vi "Scatter.vi"() -> ()   [LabVIEW 2011]
uses:
  <vilib>/Heliosphere Research LLC/Advanced Plotting Toolkit/Advanced Plotting Toolkit.lvlib
  <vilib>/Heliosphere Research LLC/Advanced Plotting Toolkit/properties/Marker_Style.ctl
  <vilib>/Heliosphere Research LLC/Advanced Plotting Toolkit/typedefs/PlotColor.ctl
  <vilib>/Heliosphere Research LLC/Advanced Plotting Toolkit/properties/Marker.ctl
  <vilib>/Heliosphere Research LLC/Advanced Plotting Toolkit/properties/Line_Style.ctl
  <vilib>/Heliosphere Research LLC/Advanced Plotting Toolkit/properties/Line.ctl
  <vilib>/Heliosphere Research LLC/Advanced Plotting Toolkit/properties/Colormap_Map.ctl
  <vilib>/Heliosphere Research LLC/Advanced Plotting Toolkit/properties/Colormap_Scaling.ctl
  <vilib>/Heliosphere Research LLC/Advanced Plotting Toolkit/properties/Colormap.ctl
  <vilib>/Heliosphere Research LLC/Advanced Plotting Toolkit/properties/Display.ctl
  <vilib>/Heliosphere Research LLC/Advanced Plotting Toolkit/api_plotting/ScatterProperties.ctl
panel:
  in  "Line Appearance":T1={"Style"=enum."Automatic", "Color"=2147483647, "Width"=nan} {"Color" items=["Automatic"=2147483647, "Black"=0, "White"=16777215, "Red"=16711680, "Green"=2263842, "Blue"=255, "Cyan"=65535, "Magenta"=16711935, "Yellow"=16776960]}
  in  "Marker Appearance":T4={"Style"=enum."Automatic", "Color"=2147483647, "Size"=nan} {"Color" items=["Automatic"=2147483647, "Black"=0, "White"=16777215, "Red"=16711680, "Green"=2263842, "Blue"=255, "Cyan"=65535, "Magenta"=16711935, "Yellow"=16776960]}
  in  "Use Colormap Values":bool=TRUE
  in  "Use Areas":bool=TRUE
  out "Log Plot":picture
  # "Scatter Plots"
  # "A scatter plot displays any data available as X/Y pairs.\n\nIn addition to simply displaying markers, Scatter.vi allows you\nto convey information using the size and color of the markers.\nThe \"Areas\" and \"Colormap Values\" inputs allow you to\ncontrol these properties on a point-by-point basis.\n\nIn this example, the areas and colors are set according to the\npoints' distance from the origin, but any 1D data may be used\ninstead.  Use the boolean controls below to turn the areas\nand colors on and off.  You can also set basic properties like the\nmarker shape and outline using the property cluster."
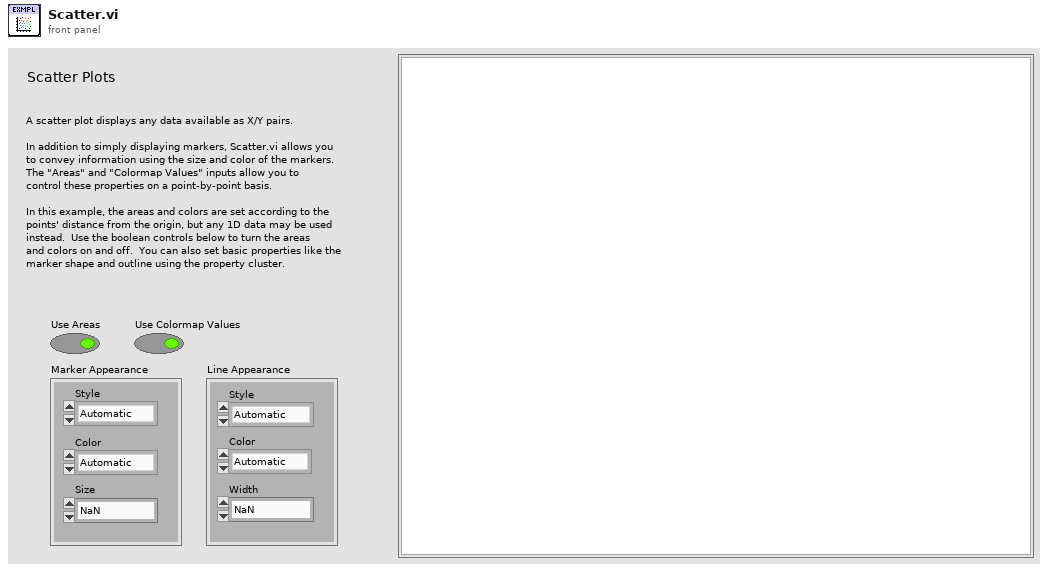
[diagram p1: front panel]
types:
  T1 = typedef "Advanced Plotting Toolkit.lvlib/Line.ctl" = cluster{"Style":T2, "Color":T3, "Width":sgl}
  T2 = typedef "Advanced Plotting Toolkit.lvlib/Line_Style.ctl" = enum16{"Automatic", "Solid", "Dashed", "Dotted", "Dash-dot", "Invisible"}
  T3 = typedef "Advanced Plotting Toolkit.lvlib/PlotColor.ctl" = u32
  T4 = typedef "Advanced Plotting Toolkit.lvlib/Marker.ctl" = cluster{"Style":T5, "Color":T3, "Size":dbl}
  T5 = typedef "Advanced Plotting Toolkit.lvlib/Marker_Style.ctl" = enum16{"Automatic", "Circle", "Square", "Triangle", "Diamond", "Star", "Invisible"}
  T6 = typedef "Advanced Plotting Toolkit.lvlib/ScatterProperties.ctl" = cluster{"Marker":T4, "Line":T1, "Colormap":T7, "Display":T10}
  T7 = typedef "Advanced Plotting Toolkit.lvlib/Colormap.ctl" = cluster{"Map":T8, "Value Min":dbl, "Value Max":dbl, "Scaling":T9, "Reverse":bool}
  T8 = typedef "Advanced Plotting Toolkit.lvlib/Colormap_Map.ctl" = enum16{"Automatic", "Rainbow", "Hot and Cold", "White-Black", "White-Blue", "White-Green", "White-Red", "Fire", "Water", "Earth", "Air", "Pastel", "Banded", "Stepped"}
  T9 = typedef "Advanced Plotting Toolkit.lvlib/Colormap_Scaling.ctl" = enum16{"Default"}
  T10 = typedef "Advanced Plotting Toolkit.lvlib/Display.ctl" = cluster{"Alpha":dbl, "Z Order":dbl}
  T11 = typedef "Advanced Plotting Toolkit.lvlib/PlotID.ctl" = i32
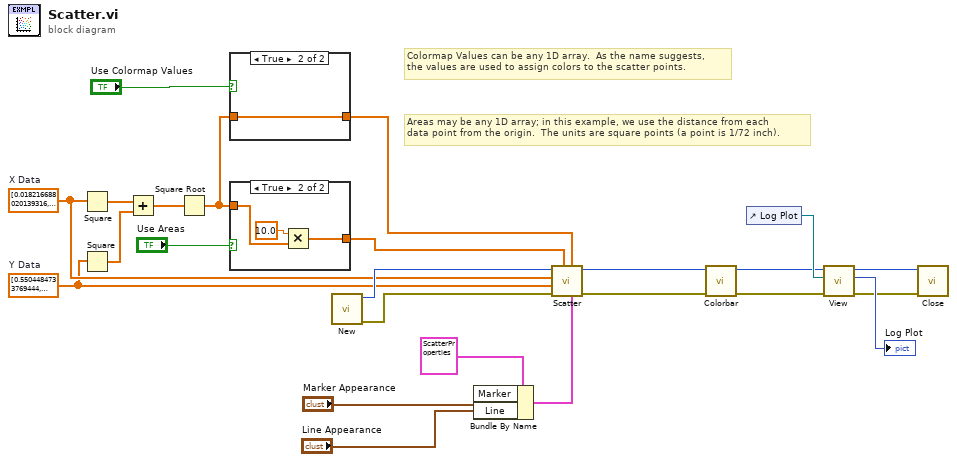
[diagram p0: block diagram]
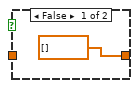
[diagram p2: hidden frame]
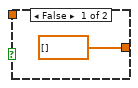
[diagram p3: hidden frame]
diagram:
  w18 = dbl[] [0.5504484733769444, 0.7340145289331643, 0.9972841843730318, 0.739103164755676, 0.4719489274133991, 0.48521359909880923, 0.268670749089941, 0.8057782296946243, 0.9028181748401577, 0.7301380893918062, 0.5945088382745651, 0.5664841888262767, 0.6245603532933975, 1.2151753773851341, 1.3751559325201912, 0.7594195233427825, 0.9174437047884547, 0.888032137496148, 1.027309928555396, 0.8465183772390145, 1.4611410254800308, 0.7854320310413877, 1.3305249271114152, 1.4337017682881403, 0.8238392444886502, 1.4695688108297478, 1.5221063546175306, 0.8713493416820589, 1.0954736948939998, 1.6983962844027416, 1.3662143684153685, 1.2125284144057185, 1.1981155398847738, 1.6763550413556394, 1.521911612001944, 1.3177646228410758, 1.413803334048454, 1.639339701921609, 1.6199879794898349, 1.68887714231835, 1.561633324060962, 1.9041851472536078, 1.3852047085256352, 1.7361658644546871, 1.699321108236791, 1.9305833477615097, 1.5819086670974714, 1.7707421705426076, 1.6307798240979468, 1.7271994646006077, 2.137995678617246, 2.522032132464089, 1.826545913354781, 2.198242909717728, 2.0516071178972615, 2.0085356605076923, 2.0475026852072133, 2.6274374789071673, 1.9588398145281822, 2.710443633941409, 2.2734091642448573, 1.9186781412150797, 2.74063295766637, 2.388394470005996, 1.965251751667286, 2.0181008951854764, 2.627408251698235, 2.7521121585893016, 2.996845074922639, 2.5235689074603425, 2.8946200153362023, 2.446783823189862, 2.693173984916524, 2.659198025424981, 2.617584433854437, 2.4731702546133696, 2.7596799615611025, 2.5173946280363584, 2.4477331523110584, 2.5605505060225764, 3.0207894708309393, 2.4943906078241262, 2.750554703670238, 3.25739696335956, 2.7696717886738034, 3.1757470969961696, 3.3922910512002282, 3.4587071311698017, 2.7460296322074402, 3.523884031785107, 3.215246060284035, 3.038415164852229, 2.876366138170591, 3.6020003032698638, 3.6666507138457884, 3.2367112464322654, 3.365310889754167, 3.225784407891871, 3.1961414172242604, 2.9919243693328026]  # Y Data
  w19 = dbl[] [0.018216688020139316, 0.6155646664152035, 0.09161887446563804, 0.5755835424122354, 0.30811405678216486, 0.9300868119887228, 0.7586483780489142, 1.089769759555441, 0.6322835384289796, 0.384787183193845, 1.2778344980742953, 0.9812998154301975, 0.3864217942054192, 1.2257226583790302, 0.5022360656236784, 1.4019622035534751, 0.6452632674815559, 0.8791971175839632, 0.8100268209069452, 1.3321489027970501, 0.6454080555060299, 1.6038888739516306, 0.9794885993611202, 1.201703057246671, 1.3700683222399341, 1.3958110923468907, 1.5420824872003653, 1.5316056401142393, 0.9179293358604258, 1.0770885097208276, 1.0840019398416834, 1.9012209722097482, 1.0103364765183542, 1.4257742799494155, 1.6657001005581127, 1.6988166953387351, 1.6494618253350257, 2.0765624770416053, 2.0856701722269166, 1.4103354500274605, 1.4609448842344637, 2.0763197759765175, 1.6784655640635633, 1.9584138400305964, 2.312762778270861, 1.5973704682789003, 2.0813213329442646, 1.9574908741379595, 2.229063128359036, 1.9824983595019636, 2.486237276605017, 2.292950981329594, 2.5449192747521874, 2.100119903850514, 1.6475780859084883, 1.8298844219321697, 2.67990510914125, 2.372726133927557, 2.347560342403799, 2.328445875817094, 2.0530610907806413, 2.675653833698585, 2.372331730832876, 2.8469250498310155, 2.0531047154397766, 2.0009313590603335, 2.4220964611753177, 2.906192593045046, 3.0335890404809187, 2.9642657046776364, 3.0534263829208763, 2.407554918793942, 2.3705271269366968, 2.5694893745920426, 2.7335864871631355, 3.2087185101465434, 2.321303978549793, 2.773069084652821, 2.5263072049612814, 3.144260339234416, 3.3009479052099295, 3.4278916561167527, 3.0928644119116417, 2.66155129272013, 2.5901214605170857, 3.073943934855988, 3.494131460204084, 3.2570294972174305, 2.7582173838209423, 3.460241818890508, 3.195976591670612, 3.220954880403231, 3.265404413183777, 3.315861959466599, 3.5414632694611354, 3.5799443170374747, 2.972322344068883, 3.301819801331183, 3.0258517262552997, 3.208561373651547]  # X Data
  # "Areas may be any 1D array; in this example, we use the distance from each\ndata point from the origin.  The units are square points (a point is 1/72 inch)."
  # "Colormap Values can be any 1D array.  As the name suggests,\nthe values are used to assign colors to the scatter points."
  n1 = Square(x=w19) -> (x^2=w17:dbl[])
  n2 = Square(x=w18) -> (x^2=w16:dbl[])
  n3 = Add(x=w17, y=w16) -> (x+y=w15:dbl[])
  n4 = Square Root(x=w15) -> (sqrt(x)=w13:dbl[])
  n5 = case shown="True" "Use Colormap Values" {
    tunnel: w13 -> [_ w26]
    tunnel: [dbl[] [] w26] -> w10
    frame False {
    }
    frame True {
    }
  }
  n6 = case shown="True" "Use Areas" {
    tunnel: w13 -> [_ w30]
    tunnel: [dbl[] [] w29] -> w11
    frame False {
    }
    frame True {
      n7 = Multiply(x=10.0, y=w30) -> (x*y=w29:dbl[])
    }
  }
  n8 = call <vilib>:"New.vi"() -> ("error out"=w20:errorcluster, "Plot ID"=w21:T11)  [unwired: 10 in]
  n9 = Bundle By Name(cluster=T6 {"Marker"={"Style"=enum."Automatic", "Color"=2147483647, "Size"=nan}, "Line"={"Style"=enum."Automatic", "Color"=2147483647, "Width"=nan}, "Colormap"={"Map"=enum."Automatic", "Value Min"=nan, "Value Max"=nan, "Scaling"=enum."Default", "Reverse"=FALSE}, "Display"={"Alpha"=nan, "Z Order"=nan}} ("Scatter Properties"), "Marker"="Marker Appearance", "Line"="Line Appearance") -> (w4:T6)
  n10 = call <vilib>:"Scatter.vi"("Properties"=w4, "Colormap Values"=w10, "Areas"=w11, "error in (no error)"=w20, "Y Data"=w18, "X Data"=w19, "Plot ID"=w21) -> ("error out"=w8:errorcluster, "Plot ID Out"=w9:T11)  [unwired: 3 in]
  n11 = call <vilib>:"Colorbar.vi"("error in (no error)"=w8, "Plot ID"=w9) -> ("error out"=w6:errorcluster, "Plot ID Out"=w7:T11)  [unwired: 8 in]
  n12 = control-ref of="Log Plot"() -> (w24:refnum<vi>)
  n13 = call <vilib>:"View.vi"("error in (no error)"=w6, "Ref for Sizing"=w24, "Plot ID"=w7) -> ("error out"=w1:errorcluster, "Picture"=→"Log Plot":picture, "Plot ID Out"=w22:T11)  [unwired: 6 in]
  n14 = call <vilib>:"Close.vi"("error in (no error)"=w1, "Plot ID"=w22) -> ()  [unwired: 9 in, 1 out]
